vi "Dashboard Main.vi"() -> ()   [LabVIEW 2013]
uses:
  <vilib>/event_ctls.llb/eventvkey.ctl
  <vilib>/Rock Robotics/WPI/Dashboard/WPI_DashboardLogging Global.vi
  <vilib>/Utility/config.llb/Write Key (String).vi
  <vilib>/Utility/config.llb/Write Key (I32).vi
  <vilib>/Utility/file.llb/Write To Spreadsheet File (DBL).vi
  <vilib>/Utility/config.llb/NI_LVConfig.lvlib
panel:
  in  "Rec Mode":enum32{"Stop", "Record", "Playback"}(radio)
  out "Image Message":string="Timeout in Camera Communications"
  in  "Dashboard Tab":T1(tab)
  out "Tension Target":dbl(slide) scale=0.0..5.0
  out "Auton":dbl
  out "Tension Adjust":dbl(slide) scale=-10.0..10.0
  in  "Camera Settings":T2={"Frame Rate"=30, "Compression"=30, "Size"=1} {"Frame Rate" scale=1.0..30.0; "Size" items=["640x480", "320x240", "160x120"]}
  out "JS1 Z":dbl(slide) scale=-1.0..1.0 scale format="%#_2e"
  out "Joystick 1":cluster{"X":dbl, "Y":dbl}[](graph)
  out "JS Buttons 1":T3
  out "JS2 Z":dbl(slide) scale=-1.0..1.0 scale format="%#_2e"
  out "Joystick 2":cluster{"X":dbl, "Y":dbl}[](graph)
  out "JS Buttons 2":T3
  out "Mode":T4(ring)=enum."Auto Disabled"
  out "Camera IP":string
  in  "DB Camera Config":bool
  out "fps":dbl format="%#.1g"
  out "Mbps":dbl format="%#.1g"
  out "Mbps 2":bool
  out "Tension":dbl(slide) scale=0.0..5.0
  out "Bottom Limit Switch":bool
  out "Top Limit Switch":bool
  out "Shooter Down":bool
  out "Arm Out":bool
  out "Upper Soft Limit":bool
  out "Low Gear?":bool
  out "Velocity":dbl
  out "Gyro Angle":dbl
  out "Lower Soft Limit":bool
  out "Ball Ready":bool
  in  "Slider 1":dbl(slide) scale=0.0..100.0
  in  "file path (dialog if empty)":path=path "C:/Users/1218/Desktop/data logs/test.txt"
  in  "Long Truss Power":dbl=2.6
  in  "Middle Truss Power":dbl=2.2
  in  "Middle Shot Power":dbl=1.95
  in  "Long Shot Power":dbl=2.05
  in  "Short Truss Power":dbl=1.75
  in  "Short Shot Power":dbl=1.56
  in  "Checkbox 2":bool
  in  "Checkbox 1":bool
  in  "Test Slider":dbl(slide) scale=0.0..100.0 scale format="%#_3g"
  in  "On/Off":bool caption="Solenoid"
  in  "Test Name":u16(ring) items=["Select the test to run...", "Example Test", "-------------------------------", "List of tests is built in robot code.", "Replace with your own automated tests."]
  in  "Test Tree":string(tree)
  in  "Motor":cluster{"Value":dbl, "Enable":bool} {"Value" scale=-1.0..1.0 scale format="%#_3g"}
  out "Progress":T5 {"Test Progress" scale=0.0..100.0}
  in  "Rev/Fwd":cluster{"Forward":bool, "Reverse":bool}
  in  "Test Ring":u16(ring) items=["Auto", "Fixed indoor", "Fixed outdoor 1", "Fixed outdoor 2", "Fixed fluorescent 1", "Fixed fluorescent 2", "Hold current"]
  in  "Listbox":i32(listbox)
  out "Tree":string(tree)
  out "Camera Image":T6(plugin-control)
  in  "Enable":bool=TRUE
  # "Customize by placing controls and indicators here and name to\nmatch Dashboard Variables on robot."
  # "This tab is a great place for autonomous settings and validation.\nCustomize by placing controls and indicators here and name to\nmatch Dashboard Variables on robot."
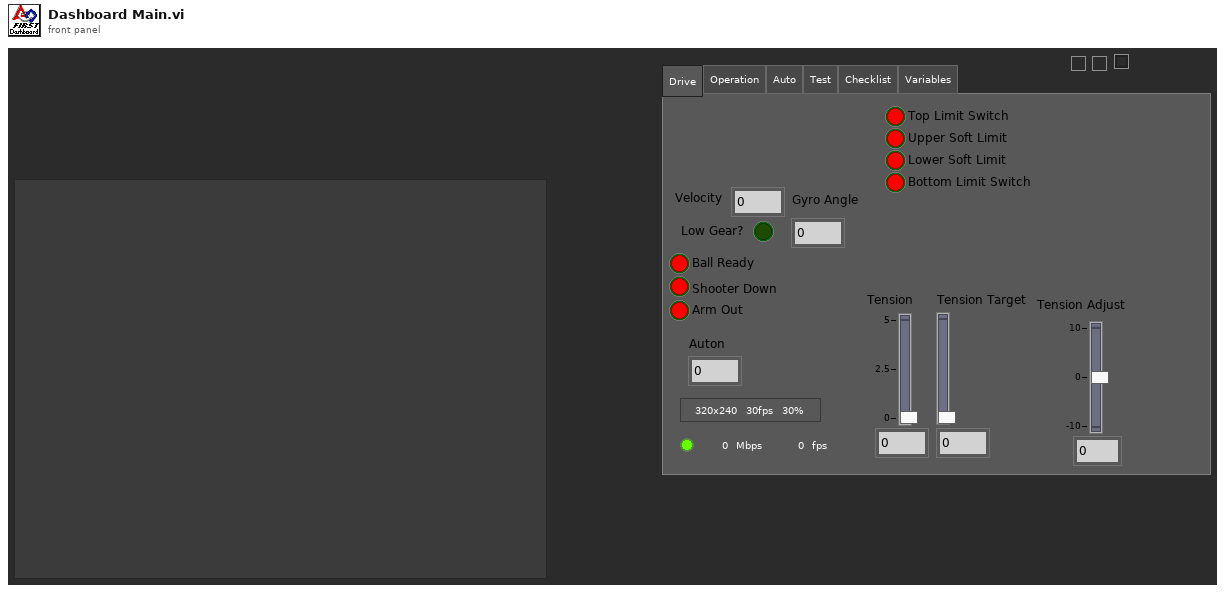
[diagram p1: front panel]
types:
  T1 = enum32{"Drive", "Operation", "Auto", "Test", "Checklist", "Variables"}
  T2 = cluster{"Frame Rate":i32, "Compression":i32, "Size":u16}
  T3 = cluster{bool, bool, bool, bool, bool, bool, bool, bool, bool, bool, bool, bool}
  T4 = enum8{"Tele-Op Disabled", "Tele-Op Enabled", "Auto Disabled", "Auto Enabled", "Test Disabled", "Test Enabled", ""}
  T5 = cluster{"Test Progress":u8, "Test Progress Text":string}
  T6 = typedef "IMAQ Image.ctl" = refnum<image>
  T7 = typedef "Image Type" = u32
  T8 = cluster{"Digital Inputs":bool[], "Digital Outputs":bool[]}
  T9 = cluster{"Competition mode":bool, "Robot Link":bool, "Autonomous":bool, "Enabled":bool, "E-Stop":bool, "Simulated":bool, "TestMode":bool, "Docked Window":bool}
  T10 = cluster{"Boolean Array[0]":bool, "Boolean Array[1]":bool, "Boolean Array[2]":bool, "Boolean Array[3]":bool, "Boolean Array[4]":bool, "Boolean Array[5]":bool, "Boolean Array[6]":bool, "Boolean Array[7]":bool, "Boolean Array[8]":bool, "Boolean Array[9]":bool, "Boolean Array[10]":bool, "Boolean Array[11]":bool}
  T11 = typedef "NI_LVConfig.lvlib/Config Data RefNum.ctl" = refnum<k1>
  T12 = typedef "eventvkey.ctl" = enum16{"ASCII", "Enter", "Return", "Shift", "Ctrl", "Alt", "Cmd", "Opt", "Caps", "NumLock", "Clear", "Break", "Up", "Down", "Left", "Right", "Insert", "Delete", "Home", "End", "PageUp", "PageDown", "Escape", "Help", "Pause", "ScrollLock", "F1", "F2", "F3", "F4", "F5", "F6", "F7", "F8", "F9", "F10", "F11", "F12", "F13", "F14", "F15", "F16", "F17", "F18", "F19", "F20", "F21", "F22", "F23", "F24", "Play", "VolumeUp", "VolumeDown", "Mute", "Two Byte Char"}
  T13 = cluster{"Image Size":bool, "Image Type":bool, "Pixel Value":bool, "ROI Information":bool, "Zoom Factor":bool}
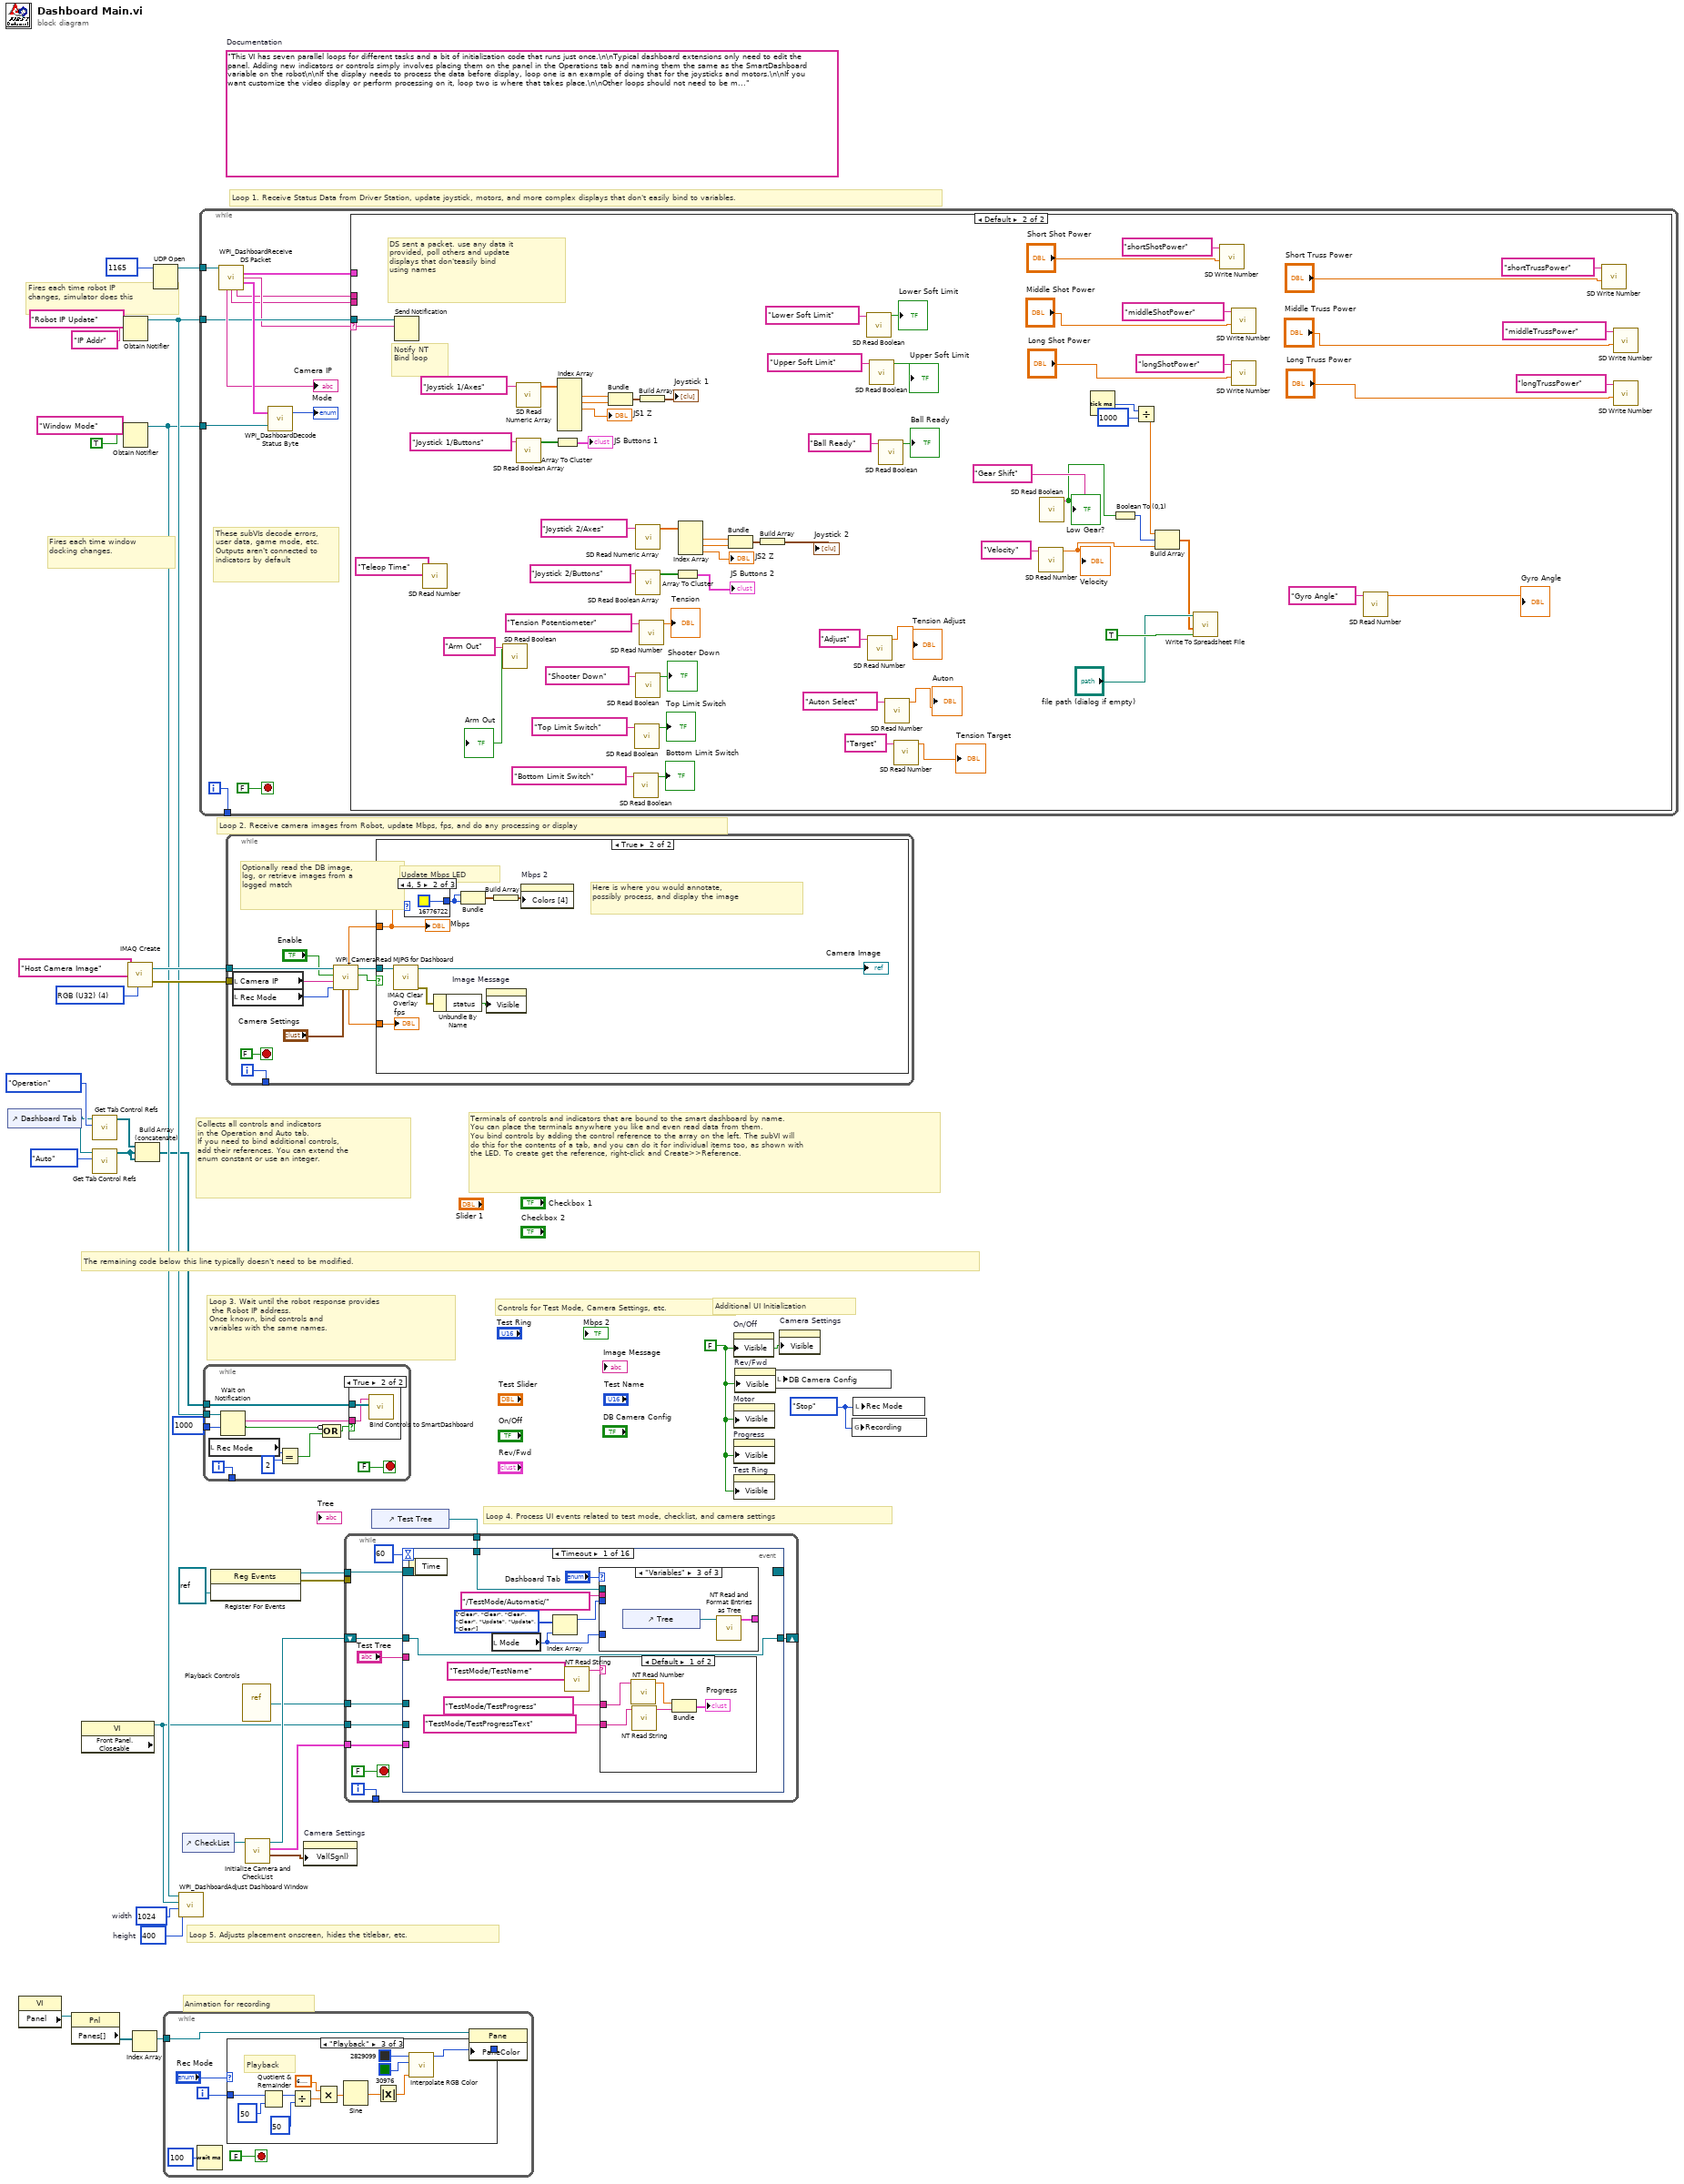
[diagram p0: block diagram]
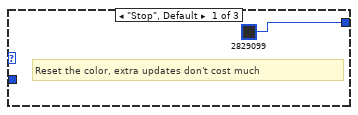
[diagram p2: hidden frame]
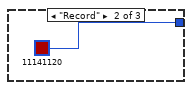
[diagram p3: hidden frame]
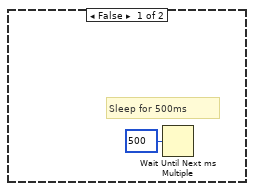
[diagram p5: hidden frame]
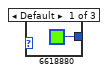
[diagram p6: hidden frame]
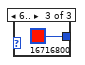
[diagram p7: hidden frame]
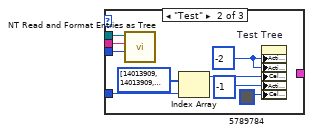
[diagram p9: hidden frame]
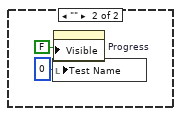
[diagram p10: hidden frame]
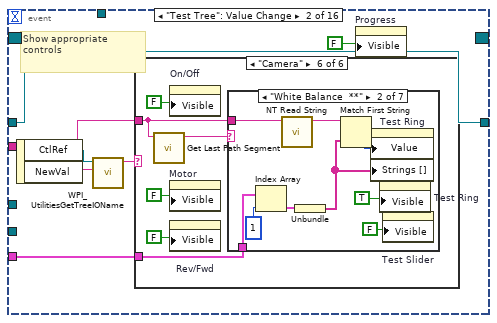
[diagram p11: hidden frame]
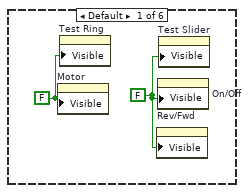
[diagram p12: hidden frame]
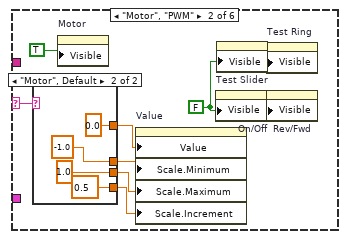
[diagram p13: hidden frame]
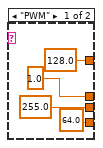
[diagram p14: hidden frame]
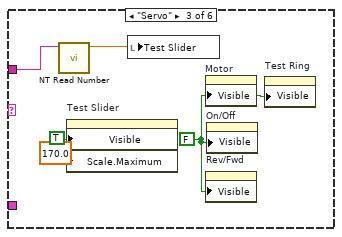
[diagram p15: hidden frame]
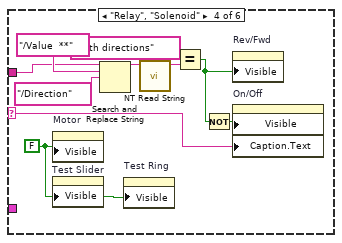
[diagram p16: hidden frame]
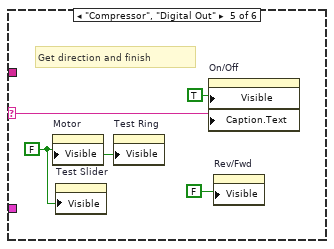
[diagram p17: hidden frame]
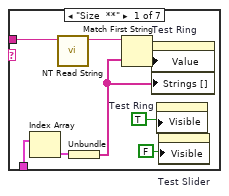
[diagram p18: hidden frame]
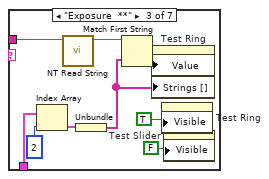
[diagram p19: hidden frame]
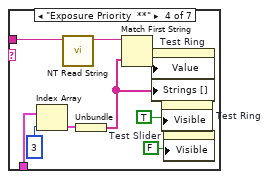
[diagram p20: hidden frame]
diagram:
  w7 = enum32{"Stop", "Record", "Playback"}."Stop" ("Rec Mode")
  w10 = 400  # height
  w11 = 1024  # width
  w24 = FALSE ("Visible")
  (unwired) "This VI has seven parallel loops for different tasks and a bit of initialization code that runs just once.\n\nTypical dashboard extensions only need to edit the panel. Adding new indicators or controls simply involves placing them on the panel in the Operations tab and naming them the same as the SmartDashboard variable on the robot\n\nIf the display needs to process the data before display, loop one is an example of doing that for the joysticks and motors.\n\nIf you want customize the video display or perform processing on it, loop two is where that takes place.\n\nOther loops should not need to be modified. They are pretty standard, and document the task they perform."  # Documentation
  w34 = T7 4 items=["Grayscale (U8)", "Grayscale (I16)", "Grayscale (SGL)", "Complex (CSG)", "RGB (U32)", "HSL (U32)", "RGB (U64)"] ("Image Type")
  # "Controls for Test Mode, Camera Settings, etc."
  # "Additional UI Initialization"
  # "Animation for recording"
  # "Fires each time robot IP\nchanges, simulator does this"
  # "Fires each time window\ndocking changes."
  # "Collects all controls and indicators\nin the Operation and Auto tab.\nIf you need to bind additional controls,\nadd their references. You can extend the\nenum constant or use an integer."
  # "The remaining code below this line typically doesn't need to be modified."
  # "Loop 4. Process UI events related to test mode, checklist, and camera settings"
  # "Terminals of controls and indicators that are bound to the smart dashboard by name.\nYou can place the terminals anywhere you like and even read data from them.\nYou bind controls by adding the control reference to the array on the left. The subVI will\ndo this for the contents of a tab, and you can do it for individual items too, as shown with\nthe LED. To create get the reference, right-click and Create>>Reference."
  # "Loop 3. Wait until the robot response provides\n the Robot IP address.\nOnce known, bind controls and\nvariables with the same names."
  # "Loop 5. Adjusts placement onscreen, hides the titlebar, etc."
  # "Loop 1. Receive Status Data from Driver Station, update joystick, motors, and more complex displays that don't easily bind to variables."
  # "Loop 2. Receive camera images from Robot, update Mbps, fps, and do any processing or display"
  n1 = control-ref of="Dashboard Tab"() -> (w5:refnum<vi>)
  n2 = property class="VI"() -> ("Panel"=w18:refnum<vi>)  [unwired: 2 in, 2 out]
  n3 = property class="Pnl"(reference=w18) -> ("Panes[]"=w19:refnum<vi>[])  [unwired: 1 in, 2 out]
  n4 = property class="VI" props=["Front Panel.Closeable"]() -> (reference out=w6:refnum<vi>)  [unwired: 2 in, 2 out]
  n5 = call <vilib>:"Get Tab Control Refs.vi"("Page Index"=T1."Operation" ("Dashboard Tab"), "TabControl in"=w5) -> ("ControlsOnPage"=w4:refnum<vi>[])  [unwired: 9 in]
  n6 = call <vilib>:"Get Tab Control Refs.vi"("Page Index"=T1."Auto" ("Dashboard Tab"), "TabControl in"=w5) -> ("ControlsOnPage"=w1:refnum<vi>[])  [unwired: 9 in]
  n7 = Obtain Notifier(name (unnamed)="Robot IP Update", notification data type="IP Addr" ("name (unnamed)")) -> (notifier out=w28:refnum<notifier>)  [unwired: 2 in, 2 out]
  n8 = Obtain Notifier(name (unnamed)="Window Mode", notification data type=TRUE) -> (notifier out=w9:refnum<notifier>)  [unwired: 2 in, 2 out]
  n9 = call "IMAQ Create"("Image Name"="Host Camera Image", "Image Type"=w34) -> ("New Image"=w32:T6, "error out"=w31:errorcluster)  [unwired: 2 in, 1 out]
  n10 = Index Array(array=w19) -> (element=w17:refnum<vi>)  [unwired: 1 in]
  n11 = Build Array (concatenate)(w4, w1, w1) -> (w3:refnum<vi>[])
  n12 = UDP Open(11:u16 1165 ("port")) -> (port=w35:refnum<k16>)  [unwired: 2 in, 4 out]
  n13 = while {
    tunnel: w17 -> [w38]
    i -> [w41]
    stop <- FALSE stop-if-true
    n14 = Wait (ms)(milliseconds to wait=u32 100) -> ()  [unwired: 1 out]
    n15 = case shown="\"Playback\"" "Rec Mode" {
      tunnel: w41 -> [_ _ w56]
      tunnel: [u32 2829099 ("Base Color") u32 11141120 ("Target Color") w45] -> w37
      frame "Stop", Default {
        # "Reset the color, extra updates don't cost much"
      }
      frame "Record" {
      }
      frame "Playback" {
        # "Playback"
        n16 = Quotient & Remainder(x=w56, y=u32 50 ("milliseconds to wait")) -> (x-y*floor(x/y)=w52:u32)  [unwired: 1 out]
        n17 = Divide(x=w52, y=u32 50 ("milliseconds to wait")) -> (x/y=w49:dbl)
        n18 = Multiply(x=6.283185307179586, y=w49) -> (x*y=w54:dbl)
        n19 = Sine(x=w54) -> (sin(x)=w53:dbl)
        n20 = Absolute Value(x=w53) -> (abs(x)=w46:dbl)
        n21 = call "Interpolate RGB Color.vi"("Proportion"=w46, "Target Color"=u32 30976, "Base Color"=u32 2829099) -> ("Result Color"=w45:u32)  [unwired: 8 in]
      }
    }
    n22 = property class="Pane"(reference=w38, "PaneColor"=w37) -> ()  [unwired: 1 in, 2 out]
  }
  n23 = call <vilib>:"WPI_DashboardAdjust Dashboard Window.vi"("height"=w10, "width"=w11, "reference in"=w6, "Notifier in"=w9) -> ()  [unwired: 8 in]
  n24 = control-ref of="CheckList"() -> (w8:refnum<vi>)
  n25 = while {
    tunnel: w35 -> [w66]
    tunnel: w28 -> [w61]
    tunnel: w9 -> [w65]
    tunnel: [w62] -> _
    i -> [w62]
    stop <- FALSE stop-if-true
    # "These subVIs decode errors, user data, game mode, etc.\nOutputs aren't connected to indicators by default"
    n26 = call <vilib>:"WPI_DashboardReceive DS Packet.vi"("Recv Socket"=w66) -> ("Driver Station"=w57:T8, "Robot IP Address"=w60:string, "Status"=w67:T9, "Camera IP Address"=→"Camera IP":string, "Low Priority User Data"=w59:string, "High Priority User Data"=w58:string)  [unwired: 1 in, 8 out]
    n27 = call <vilib>:"WPI_DashboardDecode Status Byte.vi"("Window Mode Notifier"=w65, "Status"=w67) -> ("Mode"=→"Mode":T4)  [unwired: 1 out]
    n28 = case shown="Default" w60 {
      selector: w60 -> [_ w117]
      tunnel: w61 -> [_ w118]
      tunnel: w59 -> [_ _]
      tunnel: w58 -> [_ _]
      tunnel: w57 -> [_ _]
      frame "0.0.0.0" {
        # "DS not sending packets, or no robot exists yet.\nDon't poll the variables"
      }
      frame Default {
        # "Notify NT\nBind loop"
        # "DS sent a packet. use any data it\nprovided, poll others and update\ndisplays that don'teasily bind\nusing names"
        n29 = Send Notification(notification=w117, notifier=w118) -> ()  [unwired: 1 in, 2 out]
        n30 = call <vilib>:"SD Read Number.vi"("Name"="Teleop Time") -> ()  [unwired: 8 in, 3 out]
        n31 = call <vilib>:"SD Read Boolean.vi"("Name"="Arm Out") -> ("Boolean"=→"Arm Out":bool)  [unwired: 8 in, 2 out]
        n32 = call <vilib>:"SD Read Numeric Array.vi"("Name"="Joystick 1/Axes") -> ("Numeric Array"=w134:dbl[])  [unwired: 8 in, 2 out]
        n33 = call <vilib>:"SD Read Boolean Array.vi"("Name"="Joystick 1/Buttons") -> ("Boolean Array"=w136:bool[])  [unwired: 8 in, 2 out]
        n34 = Array To Cluster(array=w136) -> (cluster=→"JS Buttons 1":T10)
        n35 = Index Array(array=w134) -> (element #1=w131:dbl, element #2=w132:dbl, element #3=→"JS1 Z":dbl)  [unwired: 6 in, 3 out]
        n36 = Bundle("Numeric"=w131, "Numeric"=w132) -> (w130:cluster{"Numeric":dbl, "Numeric":dbl})  [unwired: 1 in]
        n37 = call <vilib>:"SD Read Boolean.vi"("Name"="Bottom Limit Switch") -> ("Boolean"=→"Bottom Limit Switch":bool)  [unwired: 8 in, 2 out]
        n38 = call <vilib>:"SD Read Boolean.vi"("Name"="Top Limit Switch") -> ("Boolean"=→"Top Limit Switch":bool)  [unwired: 8 in, 2 out]
        n39 = call <vilib>:"SD Read Numeric Array.vi"("Name"="Joystick 2/Axes") -> ("Numeric Array"=w128:dbl[])  [unwired: 8 in, 2 out]
        n40 = call <vilib>:"SD Read Boolean Array.vi"("Name"="Joystick 2/Buttons") -> ("Boolean Array"=w127:bool[])  [unwired: 8 in, 2 out]
        n41 = call <vilib>:"SD Read Boolean.vi"("Name"="Shooter Down") -> ("Boolean"=→"Shooter Down":bool)  [unwired: 8 in, 2 out]
        n42 = call <vilib>:"SD Read Number.vi"("Name"="Tension Potentiometer") -> ("Numeric"=→"Tension":dbl)  [unwired: 8 in, 2 out]
        n43 = Build Array(w130) -> (→"Joystick 1":cluster{"Numeric":dbl, "Numeric":dbl}[])
        n44 = Array To Cluster(array=w127) -> (cluster=→"JS Buttons 2":T10)
        n45 = Index Array(array=w128) -> (element #1=w123:dbl, element #2=w122:dbl, element #3=→"JS2 Z":dbl)  [unwired: 3 in]
        n46 = Bundle("Numeric"=w123, "Numeric"=w122) -> (w124:cluster{"Numeric":dbl, "Numeric":dbl})  [unwired: 1 in]
        n47 = Build Array(w124) -> (→"Joystick 2":cluster{"Numeric":dbl, "Numeric":dbl}[])
        n48 = call <vilib>:"SD Read Boolean.vi"("Name"="Lower Soft Limit") -> ("Boolean"=→"Lower Soft Limit":bool)  [unwired: 8 in, 2 out]
        n49 = call <vilib>:"SD Read Number.vi"("Name"="Adjust") -> ("Numeric"=→"Tension Adjust":dbl)  [unwired: 8 in, 2 out]
        n50 = call <vilib>:"SD Read Boolean.vi"("Name"="Upper Soft Limit") -> ("Boolean"=→"Upper Soft Limit":bool)  [unwired: 8 in, 2 out]
        n51 = call <vilib>:"SD Read Boolean.vi"("Name"="Ball Ready") -> ("Boolean"=→"Ball Ready":bool)  [unwired: 8 in, 2 out]
        n52 = call <vilib>:"SD Read Number.vi"("Name"="Auton Select") -> ("Numeric"=→"Auton":dbl)  [unwired: 8 in, 2 out]
        n53 = call <vilib>:"SD Read Number.vi"("Name"="Target") -> ("Numeric"=→"Tension Target":dbl)  [unwired: 8 in, 2 out]
        n54 = call <vilib>:"SD Read Number.vi"("Name"="Velocity") -> ("Numeric"=w88:dbl)  [unwired: 8 in, 2 out]
        "Velocity" <- w88
        n55 = call <vilib>:"SD Read Boolean.vi"("Name"="Gear Shift") -> ("Boolean"=w94:bool)  [unwired: 8 in, 2 out]
        "Low Gear?" <- w94
        n56 = Tick Count (ms)() -> (millisecond timer value=w92:u32)
        n57 = Boolean To (0,1)(Boolean=w94) -> (0, 1=w89:i16)
        n58 = Divide(x=w92, y=u32 1000) -> (x/y=w90:dbl)
        n59 = Build Array(w90, w89, w88) -> (w87:dbl[])
        n60 = call-poly <vilib>:"Write To Spreadsheet File.vi"("append to file? (new file:F)"=TRUE, "1D data"=w87, "file path (dialog if empty)"="file path (dialog if empty)") -> ()  [unwired: 5 in, 1 out]
        n61 = call <vilib>:"SD Write Number.vi"("Numeric"="Short Shot Power", "Name"="shortShotPower") -> ()  [unwired: 8 in, 2 out]
        n62 = call <vilib>:"SD Write Number.vi"("Numeric"="Middle Shot Power", "Name"="middleShotPower") -> ()  [unwired: 8 in, 2 out]
        n63 = call <vilib>:"SD Write Number.vi"("Numeric"="Long Shot Power", "Name"="longShotPower") -> ()  [unwired: 8 in, 2 out]
        n64 = call <vilib>:"SD Read Number.vi"("Name"="Gyro Angle") -> ("Numeric"=→"Gyro Angle":dbl)  [unwired: 8 in, 2 out]
        n65 = call <vilib>:"SD Write Number.vi"("Numeric"="Short Truss Power", "Name"="shortTrussPower") -> ()  [unwired: 8 in, 2 out]
        n66 = call <vilib>:"SD Write Number.vi"("Numeric"="Middle Truss Power", "Name"="middleTrussPower") -> ()  [unwired: 8 in, 2 out]
        n67 = call <vilib>:"SD Write Number.vi"("Numeric"="Long Truss Power", "Name"="longTrussPower") -> ()  [unwired: 8 in, 2 out]
      }
    }
  }
  n68 = while {
    tunnel: w3 -> [w149]
    tunnel: w28 -> [w147]
    tunnel: [w145] -> _
    tunnel: u32 1000 ("milliseconds to wait") -> [w144]
    i -> [w145]
    stop <- FALSE stop-if-true
    n69 = local read "Rec Mode"() -> (w140:enum32{"Stop", "Record", "Playback"})
    n70 = Wait on Notification(notifier=w147, timeout in ms (-1)=w144) -> (notification=w146:string, timed out?=w142:bool)  [unwired: 2 in, 2 out]
    n71 = Equal?(x=w140, y=u16 2 ("Rec Mode")) -> (x = y?=w141:bool)
    n72 = Compound Arithmetic op=OR(invert w142, w141) -> (w143:bool)
    n73 = case shown="True" w143 {
      tunnel: w149 -> [_ w151]
      tunnel: w146 -> [_ w150]
      frame False {
      }
      frame True {
        n74 = call <vilib>:"Bind Controls to SmartDashboard.vi"("Bound Control Refs"=w151, "Server IP Address"=w150) -> ()  [unwired: 10 in]
      }
    }
  }
  n75 = register-events(refnum<vi> refnum) -> (reference out=w15:refnum<event-registration>, error out=w14:errorcluster)  [unwired: 2 in]
  n76 = while {
    tunnel: w32 -> [w160]
    tunnel: w31 -> [_]
    tunnel: [w161] -> _
    i -> [w161]
    stop <- FALSE stop-if-true
    # "Optionally read the DB image,\nlog, or retrieve images from a\nlogged match"
    n77 = local read "Camera IP"() -> (w153:string)
    n78 = local read "Rec Mode"() -> (w152:enum32{"Stop", "Record", "Playback"})
    n79 = call <vilib>:"WPI_CameraRead MJPG for Dashboard.vi"("Camera Settings"="Camera Settings", "Rec Mode"=w152, "Camera IP"=w153, "Enable"="Enable", "Refnum in"=w160) -> ("Active"=w157:bool, "Refnum out"=w159:T6, "FPS"=w156:dbl, "Bandwidth (Mbps)"=w155:dbl)  [unwired: 3 in]
    n80 = case shown="True" w157 {
      tunnel: w159 -> [_ w167]
      tunnel: w155 -> [_ w166]
      tunnel: w156 -> [_ w164]
      frame False {
        # "Sleep for 500ms"
        n81 = Wait Until Next ms Multiple(millisecond multiple=u32 500) -> ()  [unwired: 1 out]
      }
      frame True {
        # "Here is where you would annotate,\npossibly process, and display the image"
        # "Update Mbps LED"
        n82 = call "IMAQ Clear Overlay"("Image"=w167) -> ("error out"=w171:errorcluster, "Image Out"=→"Camera Image":T6)  [unwired: 2 in, 7 out]
        n83 = case shown="4, 5" w166 {
          tunnel: [u32 6618880 ("Color Box") u32 16776722 ("Color Box") u32 16716800 ("Color Box")] -> w168
          frame Default {
          }
          frame 4, 5 {
          }
          frame 6.. {
          }
        }
        n84 = Unbundle By Name(w171) -> ("status"=w172:bool)
        n85 = Bundle("Color Box"=w168, "Color Box"=w168) -> (w170:cluster{"Color Box":u32, "Color Box":u32})  [unwired: 1 out]
        n86 = property on="Image Message" class="Str"("Visible"=w172) -> ()  [unwired: 2 in, 2 out]
        n87 = Build Array(w170) -> (w169:cluster{"Color Box":u32, "Color Box":u32}[])
        n88 = property on="Mbps 2" class="Bool (strict)"("Colors [4]"=w169) -> ()  [unwired: 2 in, 2 out]
        "Mbps" <- w166
        "fps" <- w164
      }
    }
  }
  n89 = vi-ref "Playback Controls.vi"() -> (w16:refnum<vi>)
  n90 = call "Initialize Camera and CheckList.vi"("ListBox in"=w8) -> ("Cluster"=w22:cluster{"value":i32, "value":i32, "index":i32}, "Array"=w23:cluster{string[]}[], "File Refnum"=w21:T11)  [unwired: 8 in]
  n91 = property on="Camera Settings" class="Clust (strict)"("Val(Sgnl)"=w22) -> ()  [unwired: 2 in, 2 out]
  n92 = control-ref of="Test Tree"() -> (w20:refnum<vi>)
  n93 = while {
    tunnel: w23 -> [w183]
    shift-right: [w182] -> _
    shift-left: w21 -> [w181]
    tunnel: [w180] -> _
    tunnel: w20 -> [w179]
    tunnel: w16 -> [w178]
    tunnel: w15 -> [w177]
    tunnel: w14 -> [_]
    tunnel: w6 -> [w176]
    i -> [w180]
    stop <- FALSE stop-if-true
    n94 = event shown="[0] Timeout" {
      selector: w177 -> [_ _ _ _ _ _ _ _ _ _ _ _ _ _ _ _]
      dyn-events: [_ _ _ _ _ _ _ _ _ _ _ _ _ w421 _ _] -> _
      timeout: u32 60 ("milliseconds to wait") -> [_ _ _ _ _ _ _ _ _ _ _ _ _ _ _ _]
      tunnel: w179 -> [w193 _ _ _ _ _ _ _ _ _ _ _ _ _ _ _]
      tunnel: "Test Tree" -> [_ _ _ _ _ _ _ _ w390 w398 w400 w404 w412 _ _ _]
      tunnel: w183 -> [_ w217 _ _ _ _ w354 w384 _ _ _ _ _ _ _ _]
      tunnel: [w187 w216 w315 w320 w328 w340 w353 w377 w389 w396 w399 w403 w411 w423 w437 w438] -> w182
      tunnel: w181 -> [w187 w216 w315 w320 w328 w340 w352 w377 w389 w396 w399 w403 w411 w423 w437 w438]
      tunnel: w178 -> [_ _ _ _ _ _ _ _ _ _ _ _ _ w424 _ w441]
      tunnel: w176 -> [_ _ _ _ _ _ _ _ _ _ _ _ _ w419 _ _]
      event Timeout {
        w192 = enum16{"Update", "Clear"}[] [enum."Clear", enum."Clear", enum."Clear", enum."Clear", enum."Update", enum."Update", enum."Clear"] items=["Update", "Clear"]
        n95 = event-data() -> ()  [unwired: 1 in, 1 out]
        n96 = local read "Mode"() -> (w190:T4)
        n97 = Index Array(array=w192, index=w190) -> (element=w191:enum16{"Update", "Clear"})
        n98 = call <vilib>:"NT Read String.vi"("Name"="TestMode/TestName") -> ("String"=w196:string)  [unwired: 9 in, 1 out]
        n99 = case shown="\"Variables\"" "Dashboard Tab" {
          tunnel: w193 -> [_ w206 _]
          tunnel: "/TestMode/Automatic/" ("Name Pattern") -> [_ w205 _]
          tunnel: w191 -> [_ w204 _]
          tunnel: w190 -> [_ w202 _]
          tunnel: [_ _ w208] -> _
          frame "Operation", Default {
          }
          frame "Test" {
            w201 = -2 ("Active Item:Row Number")
            n100 = call <vilib>:"NT Read and Format Entries as Tree.vi"("Operation"=w204, "Name Pattern"=w205, "Tree Refnum"=w206) -> ()  [unwired: 7 in, 2 out]
            n101 = Index Array(array=u32[] [14013909, 14013909, 14013909, 14013909, 14013909, 16777215, 14013909], index=w202) -> (element=w200:u32)
            n102 = property on="Test Tree" class="Tree (strict)"("Active Item Row Number"=w201, "ActiveColNum"=w201, "CellBG"=w200, "Active Item Row Number"=-1 ("Active Item:Row Number"), "CellBG"=u32 5789784 ("Color Box")) -> ()  [unwired: 2 in, 2 out]
          }
          frame "Variables" {
            n103 = control-ref of="Tree"() -> (w207:refnum<vi>)
            n104 = call <vilib>:"NT Read and Format Entries as Tree.vi"("Tree Refnum"=w207) -> ("Formatted Strings"=w208:cluster{"Name":string, "Value":string}[])  [unwired: 9 in, 1 out]
          }
        }
        n105 = case shown="Default" w196 {
          tunnel: "TestMode/TestProgress" ("Name") -> [w210 _]
          tunnel: "TestMode/TestProgressText" ("Name") -> [w209 _]
          frame Default {
            n106 = call <vilib>:"NT Read Number.vi"("Name"=w210) -> ("Numeric"=w211:dbl)  [unwired: 9 in, 1 out]
            n107 = call <vilib>:"NT Read String.vi"("Name"=w209) -> ("String"=w212:string)  [unwired: 9 in, 1 out]
            n108 = Bundle("Numeric"=w211, "String"=w212) -> (→"Progress":cluster{"Numeric":dbl, "String":string})  [unwired: 1 in]
          }
          frame "" {
            n109 = local write "Test Name"(u16 0) -> ()
            n110 = property on="Progress" class="Clust (strict)"("Visible"=FALSE) -> ()  [unwired: 2 in, 2 out]
          }
        }
      }
      event "Test Tree": Value Change {
        # "Show appropriate\ncontrols"
        n111 = event-data() -> ("CtlRef"=w220:refnum<vi>, "NewVal"=w218:string)  [unwired: 1 in]
        n112 = call <vilib>:"WPI_UtilitiesGetTreeIOName.vi"("NewVal"=w218, "TreeControl in"=w220) -> ("I/O Name"=w221:string)  [unwired: 9 in]
        n113 = case shown="\"Camera\"" w221 {
          selector: w221 -> [_ w228 _ w246 w255 _]
          tunnel: w218 -> [_ _ w243 w245 _ w262]
          tunnel: w217 -> [_ _ _ _ _ w261]
          frame Default {
            w223 = FALSE ("Visible")
            w222 = FALSE ("Visible")
            n114 = property on="Motor" class="Clust (strict)"("Visible"=w222) -> ()  [unwired: 2 in, 2 out]
            n115 = property on="Test Ring" class="Ring (strict)"("Visible"=w222) -> ()  [unwired: 2 in, 2 out]
            n116 = property on="Rev/Fwd" class="Clust (strict)"("Visible"=w223) -> ()  [unwired: 2 in, 2 out]
            n117 = property on="On/Off" class="Bool (strict)"("Visible"=w223) -> ()  [unwired: 2 in, 2 out]
            n118 = property on="Test Slider" class="Slide (strict)"("Visible"=w223) -> ()  [unwired: 2 in, 2 out]
          }
          frame "Motor", "PWM" {
            w229 = FALSE ("Visible")
            n119 = case shown="\"Motor\", Default" w228 {
              tunnel: [1.0 ("Value") -1.0 ("Value")] -> w227
              tunnel: [255.0 ("Value") 1.0 ("Value")] -> w226
              tunnel: [128.0 ("Value") 0.0 ("Value")] -> w225
              tunnel: [64.0 ("Value") 0.5 ("Value")] -> w224
              frame "PWM" {
              }
              frame "Motor", Default {
              }
            }
            n120 = property on="Motor" class="Clust (strict)"("Visible"=TRUE) -> ()  [unwired: 2 in, 2 out]
            n121 = property on="Value" class="Slide (strict)"("Value"=w225, "Scale.Minimum"=w227, "Scale.Maximum"=w226, "Scale.Increment"=w224) -> ()  [unwired: 2 in, 2 out]
            n122 = property on="On/Off" class="Bool (strict)"("Visible"=w229) -> ()  [unwired: 2 in, 2 out]
            n123 = property on="Test Slider" class="Slide (strict)"("Visible"=w229) -> ()  [unwired: 2 in, 2 out]
            n124 = property on="Test Ring" class="Ring (strict)"("Visible"=w229) -> ()  [unwired: 2 in, 2 out]
            n125 = property on="Rev/Fwd" class="Clust (strict)"("Visible"=w229) -> ()  [unwired: 2 in, 2 out]
          }
          frame "Servo" {
            w241 = FALSE ("Visible")
            n126 = call <vilib>:"NT Read Number.vi"("Name"=w243) -> ("Numeric"=w242:dbl)  [unwired: 9 in, 1 out]
            n127 = property on="Test Slider" class="Slide (strict)"("Visible"=TRUE, "Scale.Maximum"=170.0 ("Scale.Range:Maximum")) -> ()  [unwired: 2 in, 2 out]
            n128 = local write "Test Slider"(w242) -> ()
            n129 = property on="Motor" class="Clust (strict)"("Visible"=w241) -> ()  [unwired: 2 in, 2 out]
            n130 = property on="Rev/Fwd" class="Clust (strict)"("Visible"=w241) -> ()  [unwired: 2 in, 2 out]
            n131 = property on="On/Off" class="Bool (strict)"("Visible"=w241) -> ()  [unwired: 2 in, 2 out]
            n132 = property on="Test Ring" class="Ring (strict)"("Visible"=w241) -> ()  [unwired: 2 in, 2 out]
          }
          frame "Relay", "Solenoid" {
            w244 = FALSE ("Visible")
            n133 = property on="Motor" class="Clust (strict)"("Visible"=w244) -> ()  [unwired: 2 in, 2 out]
            n134 = property on="Test Slider" class="Slide (strict)"("Visible"=w244) -> ()  [unwired: 2 in, 2 out]
            n135 = Search and Replace String(input string=w245, search string="/Value  **", replace string="/Direction") -> (result string=w251:string)  [unwired: 5 in, 3 out]
            n136 = property on="Test Ring" class="Ring (strict)"("Visible"=w244) -> ()  [unwired: 2 in, 2 out]
            n137 = call <vilib>:"NT Read String.vi"("Name"=w251) -> ("String"=w249:string)  [unwired: 9 in, 1 out]
            n138 = Equal?(x="Both directions", y=w249) -> (x = y?=w247:bool)
            n139 = Not(x=w247) -> (.not. x?=w248:bool)
            n140 = property on="Rev/Fwd" class="Clust (strict)"("Visible"=w247) -> ()  [unwired: 2 in, 2 out]
            n141 = property on="On/Off" class="Bool (strict)"("Visible"=w248, "Caption.Text"=w246) -> ()  [unwired: 2 in, 2 out]
          }
          frame "Compressor", "Digital Out" {
            w254 = FALSE ("Visible")
            # "Get direction and finish"
            n142 = property on="Motor" class="Clust (strict)"("Visible"=w254) -> ()  [unwired: 2 in, 2 out]
            n143 = property on="Test Slider" class="Slide (strict)"("Visible"=w254) -> ()  [unwired: 2 in, 2 out]
            n144 = property on="Test Ring" class="Ring (strict)"("Visible"=w254) -> ()  [unwired: 2 in, 2 out]
            n145 = property on="On/Off" class="Bool (strict)"("Visible"=TRUE, "Caption.Text"=w255) -> ()  [unwired: 2 in, 2 out]
            n146 = property on="Rev/Fwd" class="Clust (strict)"("Visible"=FALSE) -> ()  [unwired: 2 in, 2 out]
          }
          frame "Camera" {
            n147 = call <vilib>:"Get Last Path Segment.vi"("String in"=w262) -> ("String out"=w263:string)  [unwired: 10 in]
            n148 = property on="On/Off" class="Bool (strict)"("Visible"=FALSE) -> ()  [unwired: 2 in, 2 out]
            n149 = property on="Motor" class="Clust (strict)"("Visible"=FALSE) -> ()  [unwired: 2 in, 2 out]
            n150 = property on="Rev/Fwd" class="Clust (strict)"("Visible"=FALSE) -> ()  [unwired: 2 in, 2 out]
            n151 = case shown="\"White Balance  **\"" w263 {
              tunnel: w262 -> [w269 w278 w287 w296 w305 _ w311]
              tunnel: w261 -> [w267 w275 w284 w293 w302 _ _]
              frame "Size  **" {
                n152 = Index Array(array=w267) -> (element=w266:cluster{string[]})  [unwired: 1 in]
                n153 = call <vilib>:"NT Read String.vi"("Name"=w269) -> ("String"=w268:string)  [unwired: 9 in, 1 out]
                n154 = Unbundle(w266) -> (w264:string[])
                n155 = Match First String(2:w264, 3:w268) -> (0:w265:i32)  [unwired: 1 out]
                n156 = property on="Test Ring" class="Ring (strict)"("Value"=w265, "Strings []"=w264) -> ()  [unwired: 2 in, 2 out]
                n157 = property on="Test Ring" class="Ring (strict)"("Visible"=TRUE) -> ()  [unwired: 2 in, 2 out]
                n158 = property on="Test Slider" class="Slide (strict)"("Visible"=FALSE) -> ()  [unwired: 2 in, 2 out]
              }
              frame "White Balance  **" {
                n159 = Index Array(array=w275, index=1) -> (element=w276:cluster{string[]})
                n160 = call <vilib>:"NT Read String.vi"("Name"=w278) -> ("String"=w277:string)  [unwired: 9 in, 1 out]
                n161 = Unbundle(w276) -> (w273:string[])
                n162 = Match First String(2:w273, 3:w277) -> (0:w272:i32)  [unwired: 1 out]
                n163 = property on="Test Ring" class="Ring (strict)"("Value"=w272, "Strings []"=w273) -> ()  [unwired: 2 in, 2 out]
                n164 = property on="Test Ring" class="Ring (strict)"("Visible"=TRUE) -> ()  [unwired: 2 in, 2 out]
                n165 = property on="Test Slider" class="Slide (strict)"("Visible"=FALSE) -> ()  [unwired: 2 in, 2 out]
              }
              frame "Exposure  **" {
                n166 = Index Array(array=w284, index=2) -> (element=w285:cluster{string[]})
                n167 = call <vilib>:"NT Read String.vi"("Name"=w287) -> ("String"=w286:string)  [unwired: 9 in, 1 out]
                n168 = Unbundle(w285) -> (w281:string[])
                n169 = Match First String(2:w281, 3:w286) -> (0:w282:i32)  [unwired: 1 out]
                n170 = property on="Test Ring" class="Ring (strict)"("Value"=w282, "Strings []"=w281) -> ()  [unwired: 2 in, 2 out]
                n171 = property on="Test Ring" class="Ring (strict)"("Visible"=TRUE) -> ()  [unwired: 2 in, 2 out]
                n172 = property on="Test Slider" class="Slide (strict)"("Visible"=FALSE) -> ()  [unwired: 2 in, 2 out]
              }
              frame "Exposure Priority  **" {
                n173 = Index Array(array=w293, index=3) -> (element=w294:cluster{string[]})
                n174 = call <vilib>:"NT Read String.vi"("Name"=w296) -> ("String"=w295:string)  [unwired: 9 in, 1 out]
                n175 = Unbundle(w294) -> (w290:string[])
                n176 = Match First String(2:w290, 3:w295) -> (0:w291:i32)  [unwired: 1 out]
                n177 = property on="Test Ring" class="Ring (strict)"("Value"=w291, "Strings []"=w290) -> ()  [unwired: 2 in, 2 out]
                n178 = property on="Test Ring" class="Ring (strict)"("Visible"=TRUE) -> ()  [unwired: 2 in, 2 out]
                n179 = property on="Test Slider" class="Slide (strict)"("Visible"=FALSE) -> ()  [unwired: 2 in, 2 out]
              }
              frame "Color Enable  **" {
                n180 = Index Array(array=w302, index=4) -> (element=w303:cluster{string[]})
                n181 = call <vilib>:"NT Read String.vi"("Name"=w305) -> ("String"=w304:string)  [unwired: 9 in, 1 out]
                n182 = Unbundle(w303) -> (w299:string[])
                n183 = Match First String(2:w299, 3:w304) -> (0:w300:i32)  [unwired: 1 out]
                n184 = property on="Test Ring" class="Ring (strict)"("Value"=w300, "Strings []"=w299) -> ()  [unwired: 2 in, 2 out]
                n185 = property on="Test Ring" class="Ring (strict)"("Visible"=TRUE) -> ()  [unwired: 2 in, 2 out]
                n186 = property on="Test Slider" class="Slide (strict)"("Visible"=FALSE) -> ()  [unwired: 2 in, 2 out]
              }
              frame Default {
                n187 = property on="Test Ring" class="Ring (strict)"("Visible"=FALSE) -> ()  [unwired: 2 in, 2 out]
                n188 = property on="Test Slider" class="Slide (strict)"("Visible"=FALSE) -> ()  [unwired: 2 in, 2 out]
              }
              frame "Brightness  **", "Color Level  **", "Compression  **", "FPS  **", "Sharpness  **" {
                n189 = call <vilib>:"NT Read Number.vi"("Name"=w311) -> ("Numeric"=w310:dbl)  [unwired: 9 in, 1 out]
                n190 = local write "Test Slider"(w310) -> ()
                n191 = property on="Test Slider" class="Slide (strict)"("Visible"=TRUE, "Scale.Maximum"=100.0 ("Scale.Range:Maximum")) -> ()  [unwired: 2 in, 2 out]
                n192 = property on="Test Ring" class="Ring (strict)"("Visible"=FALSE) -> ()  [unwired: 2 in, 2 out]
              }
            }
          }
        }
        n193 = property on="Progress" class="Clust (strict)"("Visible"=FALSE) -> ()  [unwired: 2 in, 2 out]
      }
      event "Test Name": Mouse Enter {
        # "Populate the ring with the list of tests"
        n194 = event-data() -> ()  [unwired: 1 in, 1 out]
        n195 = call <vilib>:"NT Read String Array.vi"("Name"="TestMode/TestList") -> ("String Array"=w319:string[])  [unwired: 9 in, 1 out]
        n196 = Build Array (concatenate)("Select the test to run...", w319) -> (w318:string[])
        n197 = property on="Test Name" class="Ring (strict)"("Strings []"=w318) -> ()  [unwired: 2 in, 2 out]
      }
      event "Test Name": Value Change {
        w321 = FALSE ("Visible")
        # "Tell the robot the test name to run"
        n198 = event-data() -> ("NewVal"=w325:u16)  [unwired: 1 in]
        n199 = property on="Test Name" class="Ring (strict)"() -> ("Strings []"=w326:string[])  [unwired: 2 in, 2 out]
        n200 = local write "Progress"(T5 {"Test Progress"=0, "Test Progress Text"=""} ("Progress")) -> ()
        n201 = Index Array(array=w326, index=w325) -> (element=w324:string)
        n202 = call <vilib>:"NT Write String.vi"("String"=w324, "Name"="TestMode/TestName") -> ()  [unwired: 9 in, 1 out]
        n203 = property on="Progress" class="Clust (strict)"("Visible"=TRUE) -> ()  [unwired: 2 in, 2 out]
        n204 = property on="Motor" class="Clust (strict)"("Visible"=w321) -> ()  [unwired: 2 in, 2 out]
        n205 = property on="Test Slider" class="Slide (strict)"("Visible"=w321) -> ()  [unwired: 2 in, 2 out]
        n206 = property on="On/Off" class="Bool (strict)"("Visible"=w321) -> ()  [unwired: 2 in, 2 out]
        n207 = property on="Rev/Fwd" class="Clust (strict)"("Visible"=w321) -> ()  [unwired: 2 in, 2 out]
        n208 = property on="Test Ring" class="Ring (strict)"("Visible"=w321) -> ()  [unwired: 2 in, 2 out]
      }
      event "Listbox": Double Click {
        n209 = event-data() -> ("PlatMods.Shift"=w329:bool, "Row"=w331:i32)  [unwired: 1 in]
        n210 = case shown="True" w329 {
          tunnel: w331 -> [w335 _]
          tunnel: 1 -> [w334 _]
          frame False {
            n211 = property on="Listbox" class="LstBox (strict)"() -> ("Item Symbols"=w333:i32[])  [unwired: 2 in, 2 out]
            n212 = Replace Array Subset(array=w333, new element=w334, index=w335) -> (w332:i32[])
            n213 = property on="Listbox" class="LstBox (strict)"("Item Symbols"=w332) -> ()  [unwired: 2 in, 2 out]
          }
          frame True {
            w336 = 0 ("Top Row")
            n214 = property on="Listbox" class="LstBox (strict)"() -> ("Number of Rows"=w338:u32)  [unwired: 2 in, 2 out]
            n215 = Initialize Array(0, w338) -> (w337:i32[])
            n216 = property on="Listbox" class="LstBox (strict)"("Top Row"=w336, "Value"=w336, "Item Symbols"=w337) -> ()  [unwired: 2 in, 2 out]
          }
        }
      }
      event "Listbox": Key Down {
        n217 = event-data() -> ("VKey"=w342:T12)  [unwired: 1 in]
        n218 = case shown="\"Left\", \"Right\"" w342 {
          selector: w342 -> [w347 _]
          tunnel: eventvkey."Left" ("VKey") -> [w345 _]
          frame "Left", "Right" {
            n219 = Equal?(x=w345, y=w347) -> (x = y?=w346:bool)
            n220 = Select(t=0, s=w346, f=1) -> (s? t:f=w348:i32)
            n221 = property on="Listbox" class="LstBox (strict)"() -> ("Item Symbols"=w351:i32[])  [unwired: 2 in, 2 out]
            n222 = Replace Array Subset(array=w351, new element=w348, index="Listbox") -> (w350:i32[])
            n223 = property on="Listbox" class="LstBox (strict)"("Item Symbols"=w350) -> ()  [unwired: 2 in, 2 out]
          }
          frame Default {
          }
        }
      }
      event "DB Camera Config": Value Change {
        n224 = event-data() -> ("NewVal"=w355:bool)  [unwired: 1 in]
        n225 = case shown="False" w355 {
          tunnel: w354 -> [w364 _]
          tunnel: [w357 w375] -> w353
          tunnel: w352 -> [w356 w375]
          frame False {
            w371 = "Camera"
            w374 = FALSE ("Visible")
            n226 = local read "Camera Settings"() -> (w363:T2)
            n227 = Index Array(array=w364) -> (element=w367:cluster{string[]})  [unwired: 1 in]
            n228 = Unbundle(w363) -> ("Frame Rate"=w362:i32, "Compression"=w361:i32, "Size"=w365:u16)
            n229 = Unbundle(w367) -> (w366:string[])
            n230 = Index Array(array=w366, index=w365) -> (element=w360:string)
            n231 = call-poly <vilib>:"Write Key.vi"("section"=w371, "value"=w360, "key"="Size", "refnum"=w356) -> ("refnum out"=w373:T11)  [unwired: 2 in, 5 out]
            n232 = call-poly <vilib>:"Write Key.vi"("section"=w371, "value"=w362, "key"="FrameRate", "refnum"=w373) -> ("refnum out"=w372:T11)  [unwired: 1 in, 6 out]
            n233 = local write "DB Camera Config"(w374) -> ()
            n234 = property on="Camera Settings" class="Clust (strict)"("Visible"=w374) -> ()  [unwired: 2 in, 2 out]
            n235 = call-poly <vilib>:"Write Key.vi"("section"=w371, "value"=w361, "key"="Compression", "refnum"=w372) -> ("refnum out"=w358:T11)  [unwired: 1 in, 6 out]
            n236 = call <vilib>:"Close Config Data.vi"("refnum"=w358) -> ("file path"=w359:path)  [unwired: 2 in, 8 out]
            n237 = call <vilib>:"Open Config Data.vi"("configuration file path"=w359) -> ("refnum"=w357:T11)  [unwired: 8 in, 2 out]
          }
          frame True {
            n238 = property on="Camera Settings" class="Clust (strict)"("Visible"=TRUE) -> ()  [unwired: 2 in, 2 out]
          }
        }
      }
      event "Camera Settings": Value Change {
        n239 = event-data() -> ("NewVal"=w388:T2)  [unwired: 1 in]
        n240 = Index Array(array=w384) -> (element=w383:cluster{string[]})  [unwired: 1 in]
        n241 = Unbundle(w388) -> ("Frame Rate"=w379:i32, "Compression"=w378:i32, "Size"=w381:u16)
        n242 = Unbundle(w383) -> (w382:string[])
        n243 = Index Array(array=w382, index=w381) -> (element=w380:string)
        n244 = Format Into String(format string="%s   %dfps   %d%%", w380, w379, w378) -> (resulting string=w385:string)  [unwired: 2 in, 1 out]
        n245 = Build Array(w385) -> (w386:string[])
        n246 = property on="DB Camera Config" class="Bool (strict)"("Strings [4]"=w386) -> ()  [unwired: 2 in, 2 out]
      }
      event "Motor.Enable": Value Change {
        n247 = event-data() -> ("NewVal"=w394:bool)  [unwired: 1 in]
        n248 = Unbundle("Motor") -> ("Value"=w393:dbl)  [unwired: 1 out]
        n249 = Select(t=w393, s=w394, f=0.0) -> (s? t:f=w391:dbl)
        n250 = call <vilib>:"NT Write Number.vi"("Numeric"=w391, "Name"=w390) -> ()  [unwired: 9 in, 1 out]
      }
      event "Test Slider": Value Change {
        n251 = event-data() -> ("NewVal"=w397:dbl)  [unwired: 1 in]
        n252 = call <vilib>:"NT Write Number.vi"("Numeric"=w397, "Name"=w398) -> ()  [unwired: 9 in, 1 out]
      }
      event "On/Off": Value Change {
        n253 = event-data() -> ("NewVal"=w402:bool)  [unwired: 1 in]
        n254 = Boolean To (0,1)(Boolean=w402) -> (0, 1=w401:i16)
        n255 = call <vilib>:"NT Write Number.vi"("Numeric"=w401, "Name"=w400) -> ()  [unwired: 9 in, 1 out]
      }
      event "Rev/Fwd": Value Change {
        n256 = event-data() -> ("NewVal.Forward"=w410:bool, "NewVal.Reverse"=w409:bool)  [unwired: 1 in]
        n257 = Boolean To (0,1)(Boolean=w410) -> (0, 1=w406:i16)
        n258 = Boolean To (0,1)(Boolean=w409) -> (0, 1=w408:i16)
        n259 = Negate(x=w408) -> (-x=w407:i16)
        n260 = Add(x=w406, y=w407) -> (x+y=w405:i16)
        n261 = call <vilib>:"NT Write Number.vi"("Numeric"=w405, "Name"=w404) -> ()  [unwired: 9 in, 1 out]
      }
      event "Test Ring": Value Change {
        n262 = event-data() -> ("NewVal"=w414:u16)  [unwired: 1 in]
        n263 = property on="Test Ring" class="Ring (strict)"() -> ("Strings []"=w415:string[])  [unwired: 2 in, 2 out]
        n264 = Index Array(array=w415, index=w414) -> (element=w413:string)
        n265 = call <vilib>:"NT Write String.vi"("String"=w413, "Name"=w412) -> ()  [unwired: 9 in, 1 out]
      }
      event "Rec Mode": Value Change {
        # "Update globals for recording mode and path to read log from.\nClear when logging and let NetworkTables set path for vision to\nuse."
        n266 = event-data() -> ("NewVal"=w425:enum32{"Stop", "Record", "Playback"})  [unwired: 1 in]
        n267 = global write "WPI_DashboardLogging Global.vi" "Logging Filename"(path "") -> ()
        n268 = global write "WPI_DashboardLogging Global.vi" "Recording"(w425) -> ()
        n269 = case shown="\"Stop\", \"Record\"" w425 {
          tunnel: w424 -> [_ w427 w435]
          tunnel: [_ _ w434] -> w421
          tunnel: [_ _ w433] -> _
          tunnel: w419 -> [_ _ w431]
          tunnel: cluster{i32, i32} {-250, 170} -> [_ _ w430]
          tunnel: [_ _ T13 {"Image Size"=TRUE, "Image Type"=TRUE, "Pixel Value"=TRUE, "ROI Information"=TRUE, "Zoom Factor"=FALSE} ("Image Information Shown:All Elements")] -> w417
          tunnel: [_ _ TRUE ("Zoom Factor")] -> w416
          frame Default {
          }
          frame "Stop", "Record" {
            # "Place Window too"
            n270 = invoke class="VI" method="FP.Close"(reference=w427) -> (reference out=w426:refnum<vi>)  [unwired: 2 in, 2 out]
            n271 = invoke class="VI" method="Abort VI"(reference=w426) -> ()  [unwired: 2 in, 3 out]
          }
          frame "Playback" {
            n272 = call "Open Playback Panel.vi"("Offset"=w430, "DB VI Ref"=w431, "Playback in"=w435) -> ("Playback out"=w432:refnum<vi>)  [unwired: 8 in]
            n273 = register-events(w432) -> (reference out=w434:refnum<event-registration>, error out=w433:errorcluster)  [unwired: 2 in]
          }
        }
        n274 = property on="Camera Image" class="ImageControl"("Image Information Shown"=w417, "Image Information Visible"=w416) -> ()  [unwired: 2 in, 2 out]
        n275 = call <vilib>:"WPI_DashboardNT Log FieldName Cache.vi"("Operation"=enum16{"Lookup/Add", "Index", "Clear"}."Clear") -> ()  [unwired: 8 in, 3 out]
      }
      event Panel Close {
        w436 = enum32{"Stop", "Record", "Playback"}."Stop" ("Rec Mode")
        n276 = event-data() -> ()  [unwired: 1 in, 4 out]
        n277 = local write "Rec Mode"(w436) -> ()
        n278 = global write "WPI_DashboardLogging Global.vi" "Recording"(w436) -> ()
      }
      event Panel Close {
        # "Abort playback window and ourself"
        n279 = event-data() -> ()  [unwired: 1 in, 4 out]
        n280 = invoke class="VI" method="FP.Close"(reference=w441) -> (reference out=w440:refnum<vi>)  [unwired: 2 in, 2 out]
        n281 = invoke class="VI" method="Abort VI"(reference=w440) -> (error out=w439:errorcluster)  [unwired: 2 in, 2 out]
        n282 = invoke class="VI" method="Abort VI"(error in=w439) -> ()  [unwired: 2 in, 3 out]
      }
    }
  }
  n283 = property on="On/Off" class="Bool (strict)"("Visible"=w24) -> ()  [unwired: 2 in, 2 out]
  n284 = property on="Motor" class="Clust (strict)"("Visible"=w24) -> ()  [unwired: 2 in, 2 out]
  n285 = property on="Progress" class="Clust (strict)"("Visible"=w24) -> ()  [unwired: 2 in, 2 out]
  n286 = property on="Test Ring" class="Ring (strict)"("Visible"=w24) -> ()  [unwired: 2 in, 2 out]
  n287 = property on="Rev/Fwd" class="Clust (strict)"("Visible"=w24) -> ()  [unwired: 2 in, 2 out]
  n288 = local write "DB Camera Config"(w24) -> ()
  n289 = property on="Camera Settings" class="Clust (strict)"("Visible"=w24) -> ()  [unwired: 2 in, 2 out]
  n290 = global write "WPI_DashboardLogging Global.vi" "Recording"(w7) -> ()
  n291 = local write "Rec Mode"(w7) -> ()
